vi "BaseDatosEJ2.vi"() -> ()   [LabVIEW 2017]
uses:
  <vilib>/Utility/NIReport.llb/Append Text Table to Report (wrap).vi
  <vilib>/Utility/NIReport.llb/NI_report.lvclass
  <vilib>/Utility/NIReport.llb/Excel/NI_Excel.lvclass
panel:
  out "String":string
  in  "Directorio":path
  in  "Guardar":bool
  in  "Table":string[][](table)
  # "LABORATORIO DE MATERIALES"
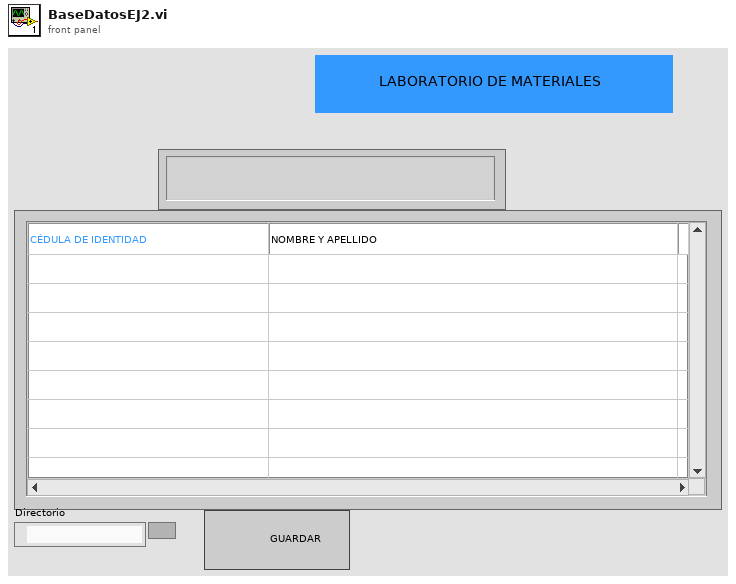
[diagram p1: front panel]
types:
  T1 = enum16{"Standard Report", "HTML", "Word", "Excel"}
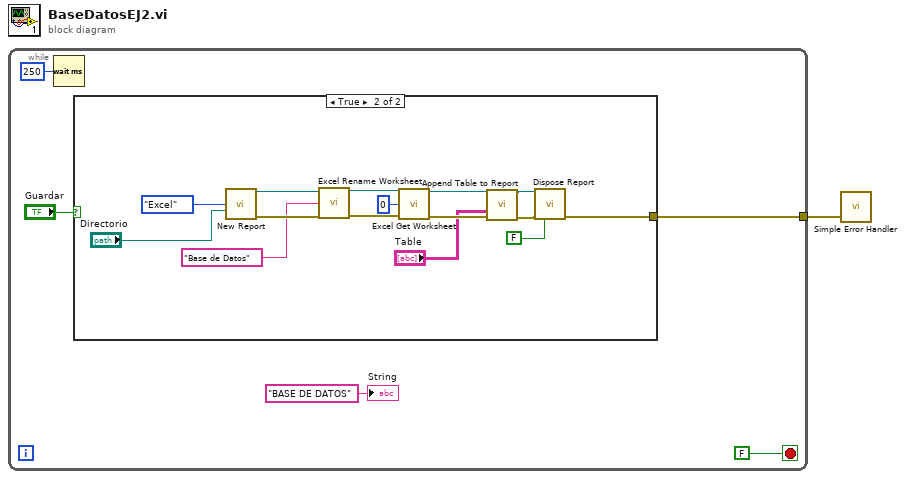
[diagram p0: block diagram]
diagram:
  n1 = while {
    tunnel: [w6] -> w1
    stop <- FALSE stop-if-true
    n2 = Wait (ms)(milliseconds to wait=u32 250) -> ()  [unwired: 1 out]
    n3 = case shown="True" "Guardar" {
      tunnel: [_ w8] -> w6
      frame False {
      }
      frame True {
        n4 = call <vilib>:"New Report.vi"("report type"=T1."Excel", "template (empty)"="Directorio") -> ("report out"=w20:refnum<class "NI_report.lvclass">, "error out"=w19:errorcluster)  [unwired: 12 in]
        n5 = call <vilib>:"Excel Rename Worksheet.vi"("report in"=w20, "worksheet name (\"\")"="Base de Datos" ("worksheet name (\"\")"), "error in (no error)"=w19) -> ("report out"=w17:refnum<class "NI_report.lvclass">, "error out"=w16:errorcluster)  [unwired: 11 in]
        n6 = call <vilib>:"Excel Get Worksheet.vi"("report in"=w17, "worksheet index (0)"=0, "error in (no error)"=w16) -> ("report out"=w14:refnum<class "NI_report.lvclass">, "error out"=w13:errorcluster)  [unwired: 11 in]
        n7 = call-poly <vilib>:"Append Table to Report.vi"("report in"=w14, "text data"="Table", "error in (no error)"=w13) -> ("report out"=w10:refnum<class "NI_report.lvclass">, "error out"=w11:errorcluster)  [unwired: 9 in, 2 out]
        n8 = call-dynamic "Dispose Report.vi"("report in"=w10, "error in (no error)"=w11, "close report? (T)"=FALSE) -> ("error out"=w8:errorcluster)  [unwired: 12 in]
      }
    }
    "String" <- "BASE DE DATOS" ("String")
  }
  n9 = call <vilib>:"Simple Error Handler.vi"("error in (no error)"=w1) -> ()  [unwired: 4 in, 5 out]
